vi "hamamatsu_initialize.vi"(0 "Camera Setup":T2={"Analog Gain (0-5)"=4, "Exposure Time"=0.01, "EM Gain (0-255)"=0, "Trigger Polarity"="ATP P", "External Trigger Mode"="ATP P", "Scan Speed"="EMD E", "External Trigger Source"="SSP H", "Scan Mode"="ESC B", "Super Pixel Binning\n(if enabled in Scan Mode)"="SMD N", "Camera Sub-array acquisition region\n(if enabled in scan mode)"={"Left"=0, "Top"=0, "Width"=0, "Height"=0}, "Use camera?"=FALSE, "# image buffers"=100, "shots per measurement"=100, "Force images to U16"=FALSE, "Low Light Sensitivity"="LLS 0", "cooling"="CSW F", "fan"="FAN F", "Frame Grabber acquisition region"={"Left"=0, "Top"=0, "Right"=0, "Bottom"=0}} {"Frame Grabber acquisition region"."Bottom" max=512 step=1; "Frame Grabber acquisition region"."Right" max=512 step=1; "Frame Grabber acquisition region"."Top" max=512 step=1; "Frame Grabber acquisition region"."Left" max=512 step=1; "shots per measurement" min=0 step=1; "# image buffers" min=0 step=1; "Camera Sub-array acquisition region\n(if enabled in scan mode)"."Height" min=16 max=512 step=16; "Camera Sub-array acquisition region\n(if enabled in scan mode)"."Width" min=16 max=512 step=16; "Camera Sub-array acquisition region\n(if enabled in scan mode)"."Top" max=496 step=16; "Camera Sub-array acquisition region\n(if enabled in scan mode)"."Left" max=496 step=16; "Analog Gain (0-5)" max=5 step=1}, 11 "error in (no error)":errorcluster) -> (3 "Image Buffers Array":T4[](array[typedef]), 4 "IMAQ Session Out":refnum<k11>, 6 "Last Valid Buffer Number":i32, 8 "Camera Temperature":dbl, 10 "number of images collected":i32, 13 "ROI":T1, 14 "Camera Acquire Settings":T3, 15 "error out":errorcluster)   [LabVIEW 2013]
uses:
  <vilib>/vision/Image Controls.llb/IMAQ Image.ctl
  Camera/Hamamatsu_C9100-13/camera_setup.ctl
  Camera/Hamamatsu_C9100-13/Hamamatsu_C9100-13.lvclass
panel:
  out "Trigger mode after IMAQ start":string
  out "Trigger mode before IMAQ Start":string
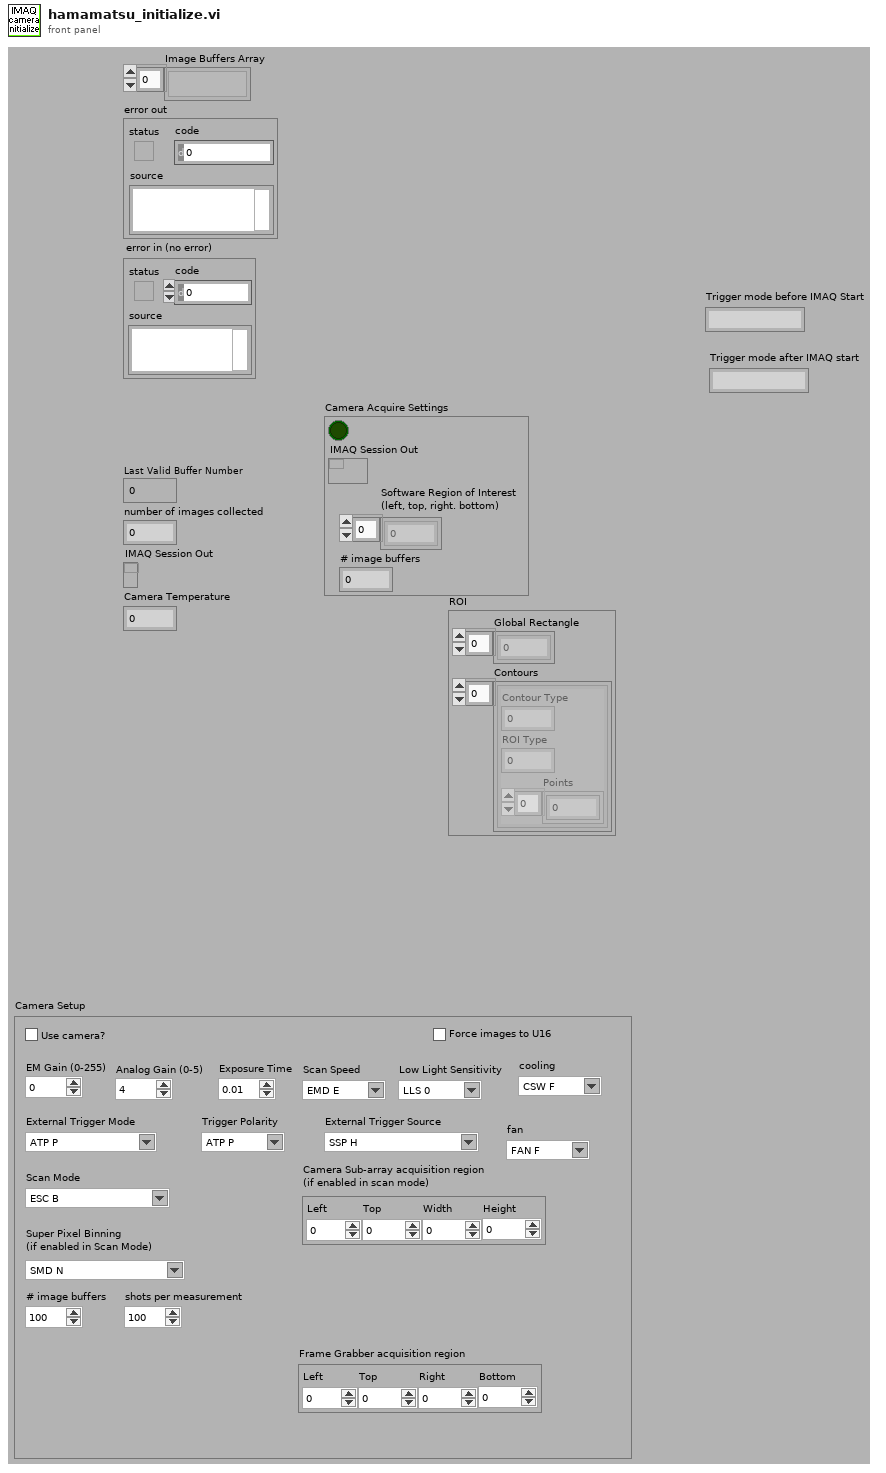
[diagram p1: front panel]
types:
  T1 = cluster{"Global Rectangle":i32[], "Contours":cluster{"Contour Type":u32, "ROI Type":u32, "Points":i32[]}[]}
  T2 = typedef "Hamamatsu_C9100-13.lvclass/camera_setup.ctl" = cluster{"Analog Gain (0-5)":u8, "Exposure Time":dbl, "EM Gain (0-255)":u8, "Trigger Polarity":string, "External Trigger Mode":string, "Scan Speed":string, "External Trigger Source":string, "Scan Mode":string, "Super Pixel Binning\n(if enabled in Scan Mode)":string, "Camera Sub-array acquisition region\n(if enabled in scan mode)":cluster{"Left":u16, "Top":u16, "Width":u16, "Height":u16}, "Use camera?":bool, "# image buffers":i32, "shots per measurement":i32, "Force images to U16":bool, "Low Light Sensitivity":string, "cooling":string, "fan":string, "Frame Grabber acquisition region":cluster{"Left":i32, "Top":i32, "Right":i32, "Bottom":i32}}
  T3 = cluster{bool, "IMAQ Session Out":refnum<k11>, "Software Region of Interest\n(left, top, right. bottom)":i32[], "# image buffers":i32}
  T4 = typedef "IMAQ Image.ctl" = refnum<image>
  T5 = cluster{"Left":u16, "Top":u16, "Width":u16, "Height":u16}
  T6 = typedef "Image Type" = u32
  T7 = cluster{bool, "IMAQ Session Out":refnum<k11>, "# image buffers":i32, "# image buffers":i32}
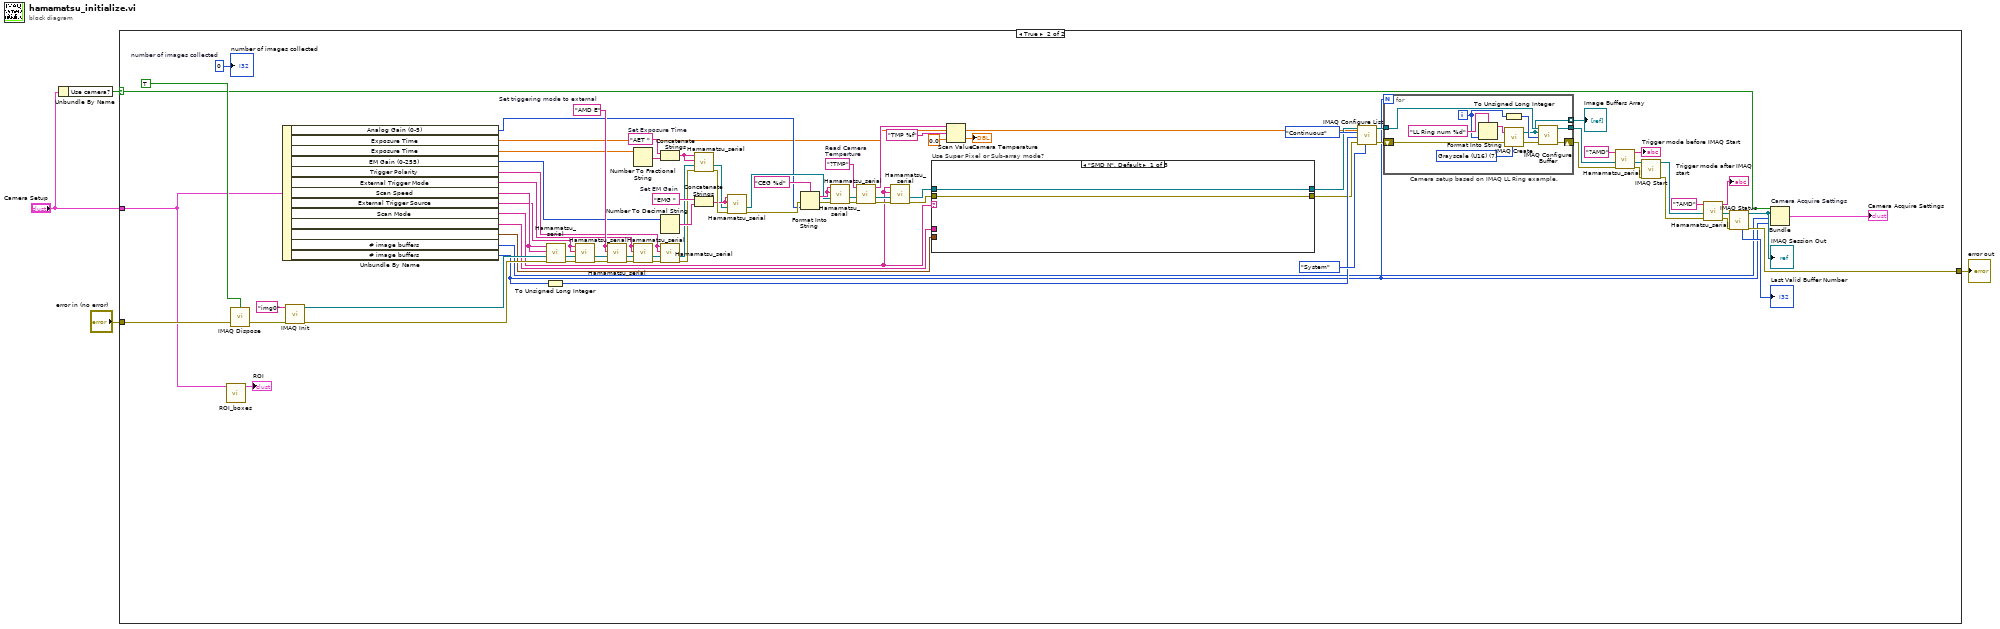
[diagram p0: block diagram]
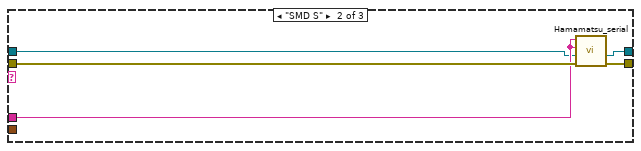
[diagram p3: hidden frame]
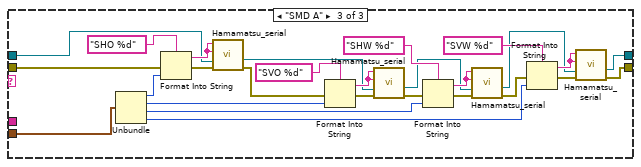
[diagram p4: hidden frame]
diagram:
  n1 = Unbundle By Name("Camera Setup") -> ("Use camera?"=w2:bool)
  n2 = case shown="True" w2 {
    selector: w2 -> [_ w43]
    tunnel: [w5 w21] -> w4
    tunnel: "error in (no error)" -> [w5 w86]
    tunnel: "Camera Setup" -> [_ w7]
    frame False {
    }
    frame True {
      w76 = "EMG "  # Set EM Gain
      w74 = "AET "  # Set Exposure Time
      w68 = "?TMP"  # Read Camera Temperture
      w65 = 0  # number of images collected
      w80 = "AMD E"  # Set triggering mode to external
      n3 = call "ROI_boxes.vi"("Camera Setup"=w7) -> ("ROI"=→"ROI":T1)  [unwired: 10 in]
      n4 = call "IMAQ Dispose"("All Images? (No)"=TRUE, "error in (no error)"=w86) -> ("error out"=w85:errorcluster)  [unwired: 4 in]
      n5 = Unbundle By Name(w7) -> ("Analog Gain (0-5)"=w20:u8, "Exposure Time"=w19:dbl, "Exposure Time"=w18:dbl, "EM Gain (0-255)"=w17:u8, "Trigger Polarity"=w16:string, "External Trigger Mode"=w15:string, "Scan Speed"=w14:string, "External Trigger Source"=w13:string, "Scan Mode"=w12:string, "Super Pixel Binning\n(if enabled in Scan Mode)"=w11:string, "Camera Sub-array acquisition region\n(if enabled in scan mode)"=w10:T5, "# image buffers"=w9:i32, "# image buffers"=w8:i32)
      n6 = call <vilib>:"IMAQ Init.vi"("error in (no error)"=w85, "Interface Name"="img0") -> ("error out"=w41:errorcluster, "IMAQ Session Out"=w50:refnum<k11>)  [unwired: 8 in]
      n7 = To Unsigned Long Integer(number=w8) -> (unsigned 32bit integer=w81:u32)
      n8 = call "Hamamatsu_serial.vi"("error in"=w41, "IMAQ Session In"=w50, "Expected Response"=w14, "Command to send"=w14) -> ("error out"=w48:errorcluster, "IMAQ Session Out"=w49:refnum<k11>)  [unwired: 5 in, 1 out]
      n9 = call "Hamamatsu_serial.vi"("error in"=w48, "IMAQ Session In"=w49, "Expected Response"=w13, "Command to send"=w13) -> ("error out"=w27:errorcluster, "IMAQ Session Out"=w28:refnum<k11>)  [unwired: 5 in, 1 out]
      n10 = call "Hamamatsu_serial.vi"("error in"=w27, "IMAQ Session In"=w28, "Expected Response"=w80, "Command to send"=w80) -> ("error out"=w25:errorcluster, "IMAQ Session Out"=w26:refnum<k11>)  [unwired: 5 in, 1 out]
      n11 = Number To Fractional String(number=w18) -> (F-format string=w75:string)  [unwired: 3 in]
      n12 = call "Hamamatsu_serial.vi"("error in"=w25, "IMAQ Session In"=w26, "Expected Response"=w15, "Command to send"=w15) -> ("error out"=w52:errorcluster, "IMAQ Session Out"=w51:refnum<k11>)  [unwired: 5 in, 1 out]
      n13 = Concatenate Strings(w74, w75) -> (w73:string)
      n14 = Number To Decimal String(number=w17) -> (decimal integer string=w78:string)  [unwired: 1 in]
      n15 = call "Hamamatsu_serial.vi"("error in"=w52, "IMAQ Session In"=w51, "Expected Response"=w16, "Command to send"=w16) -> ("error out"=w54:errorcluster, "IMAQ Session Out"=w53:refnum<k11>)  [unwired: 5 in, 1 out]
      n16 = call "Hamamatsu_serial.vi"("error in"=w54, "IMAQ Session In"=w53, "Expected Response"=w73, "Command to send"=w73) -> ("error out"=w79:errorcluster, "IMAQ Session Out"=w67:refnum<k11>)  [unwired: 5 in, 1 out]
      n17 = Concatenate Strings(w76, w78) -> (w77:string)
      n18 = call "Hamamatsu_serial.vi"("error in"=w79, "IMAQ Session In"=w67, "Expected Response"=w77, "Command to send"=w77) -> ("error out"=w58:errorcluster, "IMAQ Session Out"=w56:refnum<k11>)  [unwired: 5 in, 1 out]
      n19 = Format Into String(format string="CEG %d", error in=w58, w20) -> (resulting string=w60:string, error out=w59:errorcluster)  [unwired: 1 in]
      n20 = call "Hamamatsu_serial.vi"("error in"=w59, "IMAQ Session In"=w56, "Expected Response"=w60, "Command to send"=w60) -> ("error out"=w57:errorcluster, "IMAQ Session Out"=w55:refnum<k11>)  [unwired: 5 in, 1 out]
      n21 = call "Hamamatsu_serial.vi"("error in"=w57, "IMAQ Session In"=w55, "Command to send"=w68) -> ("error out"=w47:errorcluster, "IMAQ Session Out"=w45:refnum<k11>, "Response from Camera"=w70:string)  [unwired: 6 in]
      n22 = call "Hamamatsu_serial.vi"("error in"=w47, "IMAQ Session In"=w45, "Expected Response"=w12, "Command to send"=w12) -> ("error out"=w46:errorcluster, "IMAQ Session Out"=w44:refnum<k11>)  [unwired: 5 in, 1 out]
      n23 = case "Use Super Pixel or Sub-array mode?" shown="\"SMD N\", Default" w12 {
        tunnel: w46 -> [w89 w94 w101]
        tunnel: [w89 w93 w102] -> w63
        tunnel: [w88 w90 w103] -> w62
        tunnel: w44 -> [w88 w91 w100]
        tunnel: w11 -> [_ w92 _]
        tunnel: w10 -> [_ _ w99]
        frame "SMD N", Default {
        }
        frame "SMD S" {
          n24 = call "Hamamatsu_serial.vi"("error in"=w94, "IMAQ Session In"=w91, "Expected Response"=w92, "Command to send"=w92) -> ("error out"=w93:errorcluster, "IMAQ Session Out"=w90:refnum<k11>)  [unwired: 5 in, 1 out]
        }
        frame "SMD A" {
          n25 = Unbundle(w99) -> ("Left"=w98:u16, "Top"=w97:u16, "Width"=w96:u16, "Height"=w95:u16)
          n26 = Format Into String(format string="SHO %d", error in=w101, w98) -> (resulting string=w118:string, error out=w108:errorcluster)  [unwired: 1 in]
          n27 = call "Hamamatsu_serial.vi"("error in"=w108, "IMAQ Session In"=w100, "Expected Response"=w118, "Command to send"=w118) -> ("error out"=w109:errorcluster, "IMAQ Session Out"=w106:refnum<k11>)  [unwired: 5 in, 1 out]
          n28 = Format Into String(format string="SVO %d", error in=w109, w97) -> (resulting string=w119:string, error out=w110:errorcluster)  [unwired: 1 in]
          n29 = call "Hamamatsu_serial.vi"("error in"=w110, "IMAQ Session In"=w106, "Expected Response"=w119, "Command to send"=w119) -> ("error out"=w111:errorcluster, "IMAQ Session Out"=w105:refnum<k11>)  [unwired: 5 in, 1 out]
          n30 = Format Into String(format string="SHW %d", error in=w111, w96) -> (resulting string=w120:string, error out=w112:errorcluster)  [unwired: 1 in]
          n31 = call "Hamamatsu_serial.vi"("error in"=w112, "IMAQ Session In"=w105, "Expected Response"=w120, "Command to send"=w120) -> ("error out"=w113:errorcluster, "IMAQ Session Out"=w104:refnum<k11>)  [unwired: 5 in, 1 out]
          n32 = Format Into String(format string="SVW %d", error in=w113, w95) -> (resulting string=w121:string, error out=w114:errorcluster)  [unwired: 1 in]
          n33 = call "Hamamatsu_serial.vi"("error in"=w114, "IMAQ Session In"=w104, "Expected Response"=w121, "Command to send"=w121) -> ("error out"=w102:errorcluster, "IMAQ Session Out"=w103:refnum<k11>)  [unwired: 5 in, 1 out]
        }
      }
      n34 = Scan Value(string=w70, format string="TMP %f", default (0 dbl)=0.0 ("value (0)")) -> (value=→"Camera Temperature":dbl)  [unwired: 1 out]
      n35 = call <vilib>:"IMAQ Configure List.vi"("Memory Location"=enum16{"System", "Onboard"}."System", "Region of interest"=w19, "error in (no error)"=w63, "Number of buffers"=w81, "Continuous?"=enum16{"One-Shot", "Continuous"}."Continuous", "IMAQ Session In"=w62) -> ("error out"=w23:errorcluster, "IMAQ Session Out"=w24:refnum<k11>)  [unwired: 4 in]
      n36 = for "Camera setup based on IMAQ LL Ring example." {
        N: w8 -> [_]
        tunnel: [w132] -> w36
        tunnel: w24 -> [w130]
        shift-right: [w127] -> w38
        shift-left: w23 -> [w131]
        tunnel: [w122] -> w64 mode=indexing
        i -> [w125]
        w126 = T6 7 items=["Grayscale (U8)", "Grayscale (I16)", "Grayscale (SGL)", "Complex (CSG)", "RGB (U32)", "HSL (U32)", "RGB (U64)", "Grayscale (U16)"] ("Image Type")
        n37 = Format Into String(format string="LL Ring num %d", w125) -> (resulting string=w129:string)  [unwired: 2 in, 1 out]
        n38 = To Unsigned Long Integer(number=w125) -> (unsigned 32bit integer=w124:u32)
        n39 = call "IMAQ Create"("Image Name"=w129, "Image Type"=w126, "error in (no error)"=w131) -> ("New Image"=w122:T4, "error out"=w123:errorcluster)  [unwired: 2 in]
        n40 = call <vilib>:"IMAQ Configure Buffer.vi"("error in (no error)"=w123, "Buffer Number"=w124, "Image In"=w122, "IMAQ Session In"=w130) -> ("error out"=w127:errorcluster, "IMAQ Session Out"=w132:refnum<k11>)  [unwired: 6 in]
      }
      "Image Buffers Array" <- w64
      n41 = call "Hamamatsu_serial.vi"("error in"=w38, "IMAQ Session In"=w36, "Command to send"="?AMD") -> ("error out"=w37:errorcluster, "IMAQ Session Out"=w29:refnum<k11>, "Response from Camera"=→"Trigger mode before IMAQ Start":string)  [unwired: 6 in]
      n42 = call <vilib>:"IMAQ Start.vi"("error in (no error)"=w37, "IMAQ Session In"=w29) -> ("error out"=w33:errorcluster, "IMAQ Session Out"=w31:refnum<k11>)  [unwired: 8 in]
      n43 = call "Hamamatsu_serial.vi"("error in"=w33, "IMAQ Session In"=w31, "Command to send"="?AMD") -> ("error out"=w32:errorcluster, "IMAQ Session Out"=w30:refnum<k11>, "Response from Camera"=→"Trigger mode after IMAQ start":string)  [unwired: 6 in]
      n44 = call <vilib>:"IMAQ Status.vi"("error in (no error)"=w32, "IMAQ Session In"=w30) -> ("error out"=w21:errorcluster, "IMAQ Session Out"=w22:refnum<k11>, "Last Valid Buffer Number"=→"Last Valid Buffer Number":i32)  [unwired: 5 in, 2 out]
      "IMAQ Session Out" <- w22
      n45 = Bundle "Camera Acquire Settings"(w43, "IMAQ Session Out"=w22, "# image buffers"=w9, "# image buffers"=w8) -> (→"Camera Acquire Settings":T7)  [unwired: 1 in]
      "number of images collected" <- w65
    }
  }
  "error out" <- w4
